vi "第一个LabVIEW例子.vi"() -> ()   [LabVIEW 2018]
panel:
  in  "停止":bool
  out "进度条控制":u8(slide) scale=0.0..100.0
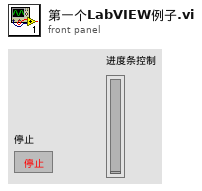
[diagram p1: front panel]
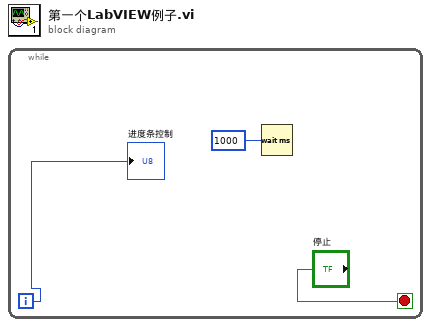
[diagram p0: block diagram]
diagram:
  n1 = while {
    i -> [w2]
    stop <- "停止" stop-if-true
    n2 = Wait (ms)(milliseconds to wait=u32 1000 ("毫秒计时值")) -> ()  [unwired: 1 out]
    "进度条控制" <- w2
  }
